vi "Delete Instance Data.vi"(0 "Data Array":T1[](array[typedef]), 5 "Cell String":string, 11 "Error In":errorcluster) -> (4 "Data Array Out":T1[](array[typedef]), 15 "Error Out":errorcluster)   [LabVIEW 2021, in "Calculator.lvlib"]
doc: "This VI checks for the instance in data array and deletes it."
uses:
  Calculator.lvlib
  Classes/NumericOperation/NumericOperation.lvclass
  Controls/Class Data.ctl
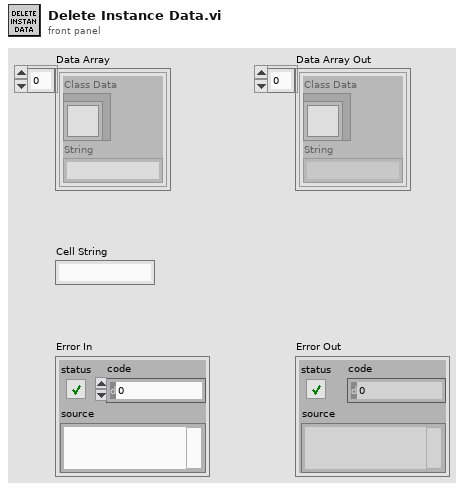
[diagram p1: front panel]
types:
  T1 = typedef "Calculator.lvlib/Class Data.ctl" = cluster{"Class Data":refnum<class "NumericOperation.lvclass">, "String":string}
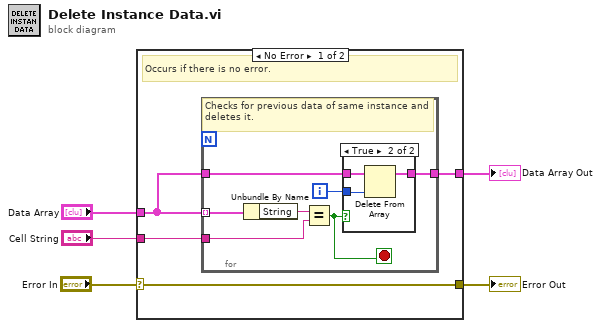
[diagram p0: block diagram]
diagram:
  n1 = case shown="No Error" "Error In" {
    selector: "Error In" -> [w6 w22]
    tunnel: "Cell String" -> [w9 _]
    tunnel: "Data Array" -> [w8 w21]
    tunnel: [w7 w21] -> w3
    tunnel: [w6 w22] -> w1
    frame No Error {
      # "Occurs if there is no error."
      n2 = for {
        tunnel: w8 -> [w14] mode=indexing
        tunnel: w9 -> [w12]
        tunnel: w8 -> [w11]
        tunnel: [w10] -> w7
        i -> [w16]
        stop <- w15 stop-if-true
        # "Checks for previous data of same instance and deletes it."
        n3 = Unbundle By Name(w14) -> ("String"=w13:string)
        n4 = Equal?(x=w13, y=w12) -> (x = y?=w15:bool)
        n5 = case shown="True" w15 {
          tunnel: w16 -> [_ w20]
          tunnel: w11 -> [w17 w19]
          tunnel: [w17 w18] -> w10
          frame False {
          }
          frame True {
            n6 = Delete From Array(array=w19, index=w20) -> (array with subset deleted=w18:T1[])  [unwired: 1 in, 1 out]
          }
        }
      }
    }
    frame Error {
      # "Occurs if there is error."
    }
  }
  "Data Array Out" <- w3
  "Error Out" <- w1
